vi "SavePrevAcqRunState.vi"(8 "error in (no error)":errorcluster, 11 "S4GUI in":refnum<class "S4GUI.lvclass">) -> (0 "error out":errorcluster, 3 "S4GUI out":refnum<class "S4GUI.lvclass">)   [LabVIEW 2018, in "S4GUI.lvclass"]
uses:
  S4GUI.lvclass
  S4GUI.lvclass/S4GUI.ctl
  Acquisition/Acquisition.lvclass
  Channel/Channel.lvclass
  StateMachine/State Machine.lvclass
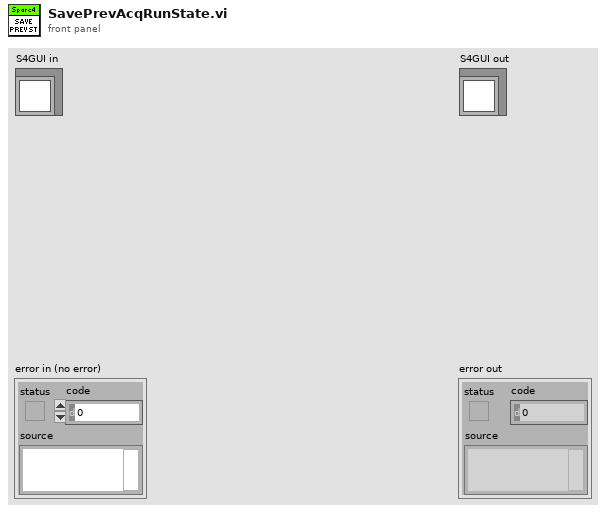
[diagram p1: front panel]
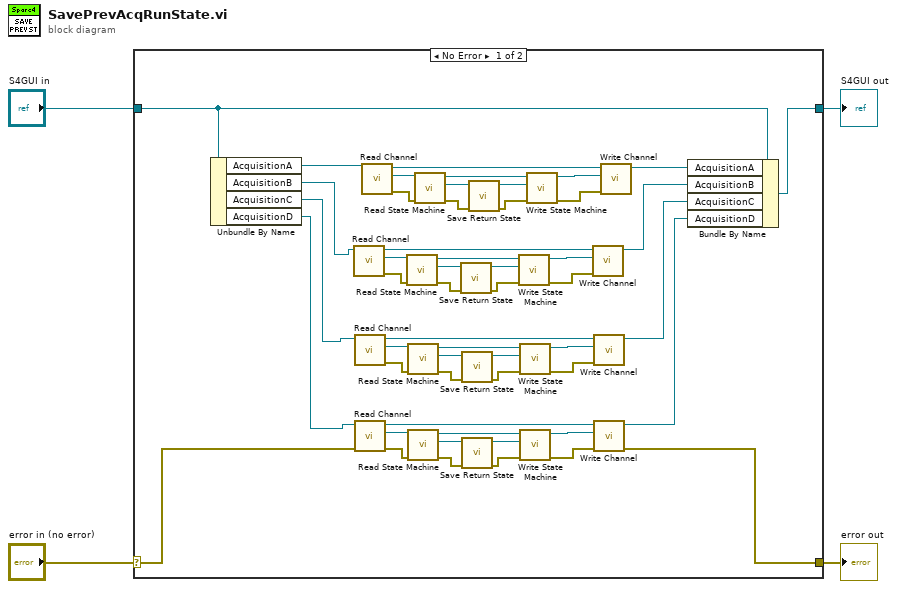
[diagram p0: block diagram]
diagram:
  n1 = case shown="No Error" "error in (no error)" {
    selector: "error in (no error)" -> [w6 w58]
    tunnel: [w5 w58] -> w3
    tunnel: [w43 w57] -> w1
    tunnel: "S4GUI in" -> [w45 w57]
    frame No Error {
      n2 = Unbundle By Name(w45) -> ("AcquisitionA"=w56:refnum<class "Acquisition.lvclass">, "AcquisitionB"=w10:refnum<class "Acquisition.lvclass">, "AcquisitionC"=w11:refnum<class "Acquisition.lvclass">, "AcquisitionD"=w12:refnum<class "Acquisition.lvclass">)
      n3 = call-dynamic "Read Channel.vi"("Acquisition in"=w10) -> ("error out"=w40:errorcluster, "Channel.lvclass"=w42:refnum<class "Channel.lvclass">, "Acquisition out"=w36:refnum<class "Acquisition.lvclass">)  [unwired: 8 in]
      n4 = call-dynamic "Read Channel.vi"("Acquisition in"=w11) -> ("error out"=w30:errorcluster, "Channel.lvclass"=w32:refnum<class "Channel.lvclass">, "Acquisition out"=w26:refnum<class "Acquisition.lvclass">)  [unwired: 8 in]
      n5 = call-dynamic "Read Channel.vi"("error in (no error)"=w6, "Acquisition in"=w12) -> ("error out"=w20:errorcluster, "Channel.lvclass"=w22:refnum<class "Channel.lvclass">, "Acquisition out"=w16:refnum<class "Acquisition.lvclass">)  [unwired: 7 in]
      n6 = call-dynamic "Read Channel.vi"("Acquisition in"=w56) -> ("error out"=w53:errorcluster, "Channel.lvclass"=w55:refnum<class "Channel.lvclass">, "Acquisition out"=w49:refnum<class "Acquisition.lvclass">)  [unwired: 8 in]
      n7 = call-dynamic "Read State Machine.vi"("error in (no error)"=w40, "Device in"=w42) -> ("error out"=w39:errorcluster, "State Machine.lvclass"=w41:refnum<class "State Machine.lvclass">, "Device out"=w37:refnum<class "Channel.lvclass">)  [unwired: 7 in]
      n8 = call-dynamic "Read State Machine.vi"("error in (no error)"=w30, "Device in"=w32) -> ("error out"=w29:errorcluster, "State Machine.lvclass"=w31:refnum<class "State Machine.lvclass">, "Device out"=w27:refnum<class "Channel.lvclass">)  [unwired: 7 in]
      n9 = call-dynamic "Read State Machine.vi"("error in (no error)"=w20, "Device in"=w22) -> ("error out"=w19:errorcluster, "State Machine.lvclass"=w21:refnum<class "State Machine.lvclass">, "Device out"=w17:refnum<class "Channel.lvclass">)  [unwired: 7 in]
      n10 = call-dynamic "Read State Machine.vi"("error in (no error)"=w53, "Device in"=w55) -> ("error out"=w52:errorcluster, "State Machine.lvclass"=w54:refnum<class "State Machine.lvclass">, "Device out"=w50:refnum<class "Channel.lvclass">)  [unwired: 7 in]
      n11 = call-dynamic "Save Return State.vi"("error in (no error)"=w39, "State Machine in"=w41) -> ("error out"=w33:errorcluster, "State Machine out"=w38:refnum<class "State Machine.lvclass">)  [unwired: 8 in]
      n12 = call-dynamic "Save Return State.vi"("error in (no error)"=w29, "State Machine in"=w31) -> ("error out"=w23:errorcluster, "State Machine out"=w28:refnum<class "State Machine.lvclass">)  [unwired: 8 in]
      n13 = call-dynamic "Save Return State.vi"("error in (no error)"=w19, "State Machine in"=w21) -> ("error out"=w13:errorcluster, "State Machine out"=w18:refnum<class "State Machine.lvclass">)  [unwired: 8 in]
      n14 = call-dynamic "Save Return State.vi"("error in (no error)"=w52, "State Machine in"=w54) -> ("error out"=w46:errorcluster, "State Machine out"=w51:refnum<class "State Machine.lvclass">)  [unwired: 8 in]
      n15 = call-dynamic "Write State Machine.vi"("error in (no error)"=w33, "State Machine.lvclass"=w38, "Device in"=w37) -> ("error out"=w35:errorcluster, "Device out"=w34:refnum<class "Channel.lvclass">)  [unwired: 7 in]
      n16 = call-dynamic "Write State Machine.vi"("error in (no error)"=w23, "State Machine.lvclass"=w28, "Device in"=w27) -> ("error out"=w25:errorcluster, "Device out"=w24:refnum<class "Channel.lvclass">)  [unwired: 7 in]
      n17 = call-dynamic "Write State Machine.vi"("error in (no error)"=w13, "State Machine.lvclass"=w18, "Device in"=w17) -> ("error out"=w15:errorcluster, "Device out"=w14:refnum<class "Channel.lvclass">)  [unwired: 7 in]
      n18 = call-dynamic "Write State Machine.vi"("error in (no error)"=w46, "State Machine.lvclass"=w51, "Device in"=w50) -> ("error out"=w48:errorcluster, "Device out"=w47:refnum<class "Channel.lvclass">)  [unwired: 7 in]
      n19 = call-dynamic "Write Channel.vi"("error in (no error)"=w35, "Channel.lvclass"=w34, "Acquisition in"=w36) -> ("Acquisition out"=w9:refnum<class "Acquisition.lvclass">)  [unwired: 7 in, 1 out]
      n20 = call-dynamic "Write Channel.vi"("error in (no error)"=w25, "Channel.lvclass"=w24, "Acquisition in"=w26) -> ("Acquisition out"=w8:refnum<class "Acquisition.lvclass">)  [unwired: 7 in, 1 out]
      n21 = call-dynamic "Write Channel.vi"("error in (no error)"=w15, "Channel.lvclass"=w14, "Acquisition in"=w16) -> ("error out"=w5:errorcluster, "Acquisition out"=w7:refnum<class "Acquisition.lvclass">)  [unwired: 7 in]
      n22 = call-dynamic "Write Channel.vi"("error in (no error)"=w48, "Channel.lvclass"=w47, "Acquisition in"=w49) -> ("Acquisition out"=w44:refnum<class "Acquisition.lvclass">)  [unwired: 7 in, 1 out]
      n23 = Bundle By Name(cluster=w45, "AcquisitionA"=w44, "AcquisitionB"=w9, "AcquisitionC"=w8, "AcquisitionD"=w7) -> (w43:refnum<class "S4GUI.lvclass">)
    }
    frame Error {
    }
  }
  "error out" <- w3
  "S4GUI out" <- w1
